vi "AE DICOM.vi"(7 "Action":T1, 8 "Error In":errorcluster) -> (0 "Error Out":errorcluster)   [LabVIEW 2013, in "main.lvlib"]
uses:
  main.lvlib
  Controls/Enum DICOM.ctl
  Controls/Enum Save Action Events.ctl
  Controls/Enum Variables.ctl
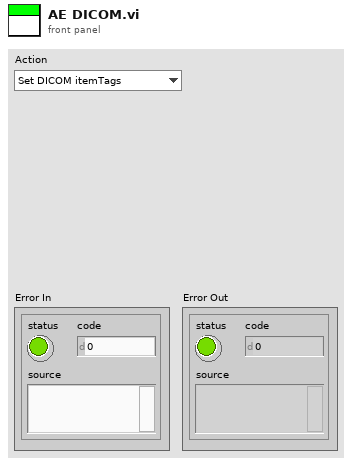
[diagram p1: front panel]
types:
  T1 = typedef "main.lvlib/Enum DICOM.ctl" = enum16{"Set DICOM itemTags", "Set Dicom Encoding", "Set DICOM Attributes"}
  T2 = typedef "main.lvlib/Enum Variables.ctl" = enum16{"SetAcqFilter", "GetAcqFilter", "Set Filter", "Get Filter", "Set Height", "Get Height", "Set Recorded Height", "Get Recorded Height", "Set Blue Pressure", "Get Blue Pressure", "Set Red Pressure", "Get Red Pressure", "Init", "Reset Pressure", "Set Red Cursors", "Get Red Cursors", "Set Blue Cursors", "Get Blue Cursors", "Set Language", "Get Language", "Set Active Graphs", "Get ActiveGraphs", "Set Method", "Get Method", "Set Encryption", "Get Encryption", "Set ExcelVersion", "Get ExcelVersion", "Set DICOM Avail", "Get DICOM Avail", "Set DICOM Encode", "Get DICOM Encode", "Set JournalExport", "Get JournalExport", "Set Sequence", "Get Sequence", "Set DAQ Connected", "Get DAQ Connected", "Set Current Graph", "Get Current Graph", "Set General Settings", "Get Hyphenation", "Set Arm Calc Method", "Get Arm Calc Method", "Set Dicom Tags", "Get Dicom Tags", "Set BT Serial", "Get BT Serial", "Set BT Accepted Serials", "Get BT Accepted Serials", "Get BT License", "Set BT License"}
  T3 = typedef "main.lvlib/Enum Save Action Events.ctl" = enum16{"LoadReportPath", "SaveReportPath", "Load Graph Path", "Save Graph Path", "LoadDataPath", "SaveDataPath", "Load Template Path", "Save Template Path", "Load PressureFactor", "Save PressureFactor", "Init", "Load Listbox", "Save Listbox", "LoadHospInfo", "SaveHospInfo", "Load DICOM Activation", "Save DICOM Activation", "LoadDICOMInfoWL", "SaveDICOMInfoWL", "LoadDICOMInfoPACS", "SaveDICOMInfoPACS", "Load ArmCalcMethod", "Save ArmCalcMethod", "LoadItemTags", "SaveItemTags", "LoadDICOMEncoding", "SaveDICOMEncoding", "LoadJournalType", "SaveJournalType", "LoadAcqFilterType", "SaveAcqFilterType", "Load Sequence", "Save Sequence", "Load Acquisition Mode", "Save Acquisition Mode", "Load General Settings", "Save General Settings", "Load Language", "Save Language", "Load Dicom Tags", "Save Dicom Tags", "Load BT Serial", "Save BT Serial", "Load BT License", "Save BT License"}
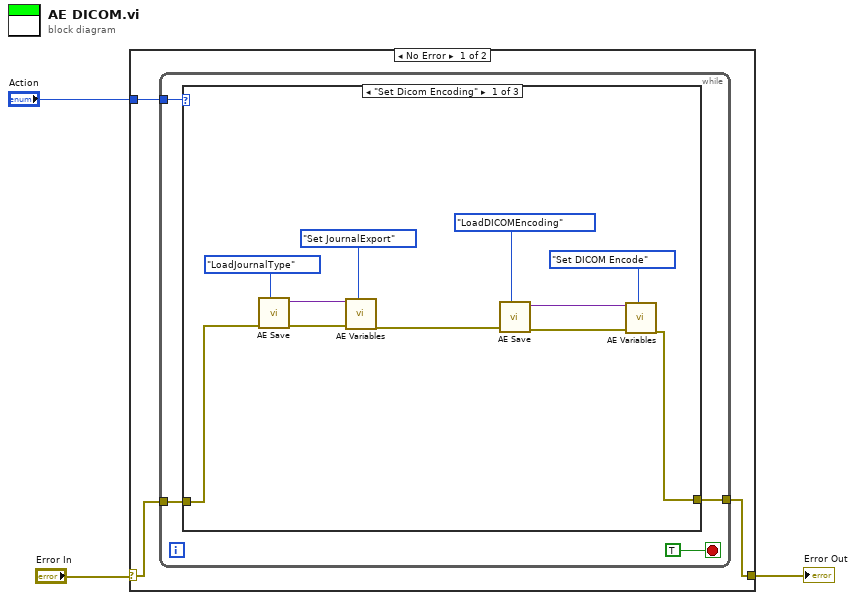
[diagram p0: block diagram]
diagram:
  n1 = case shown="No Error" "Error In" {
    selector: "Error In" -> [w5 w24]
    tunnel: "Action" -> [w6 _]
    tunnel: [w4 w24] -> w1
    frame No Error {
      n2 = while {
        tunnel: w6 -> [w10]
        tunnel: w5 -> [w8]
        tunnel: [w7] -> w4
        stop <- TRUE stop-if-true
        n3 = case shown="\"Set Dicom Encoding\"" w10 {
          tunnel: w8 -> [w15 w22 w23]
          tunnel: [w17 w22 w23] -> w7
          frame "Set Dicom Encoding" {
            n4 = call "AE Save.vi"("error in (no error)"=w15, "Action"=Enum_Save_Action_Events."LoadJournalType") -> ("error out"=w12:errorcluster, "Anything"=w13:variant)  [unwired: 7 in]
            n5 = call "AE Variables.vi"("VariantIn"=w13, "error in (no error)"=w12, "Action"=Enum_Variables."Set JournalExport") -> ("error out"=w11:errorcluster)  [unwired: 9 in, 7 out]
            n6 = call "AE Save.vi"("error in (no error)"=w11, "Action"=Enum_Save_Action_Events."LoadDICOMEncoding") -> ("error out"=w20:errorcluster, "Anything"=w19:variant)  [unwired: 7 in]
            n7 = call "AE Variables.vi"("VariantIn"=w19, "error in (no error)"=w20, "Action"=Enum_Variables."Set DICOM Encode") -> ("error out"=w17:errorcluster)  [unwired: 9 in, 7 out]
          }
          frame "Set DICOM Attributes" {
          }
          frame "Set DICOM itemTags" {
          }
        }
      }
    }
    frame Error {
    }
  }
  "Error Out" <- w1
